vi "Save Config File (to internal memory).vi"(8 "error in (no error)":errorcluster, 10 "Name of the config to store in the DAS":string, 11 "VISA resource name":refnum<visa-resource-name>) -> (0 "error out":errorcluster, 3 "VISA resource name out":refnum<visa-resource-name>)   [LabVIEW 2017, in "Sefram DAS220.lvlib"]
doc: "Save the current configuration into the device internal memory."
uses:
  <instrlib>/Sefram DAS220/Sefram DAS220.lvlib
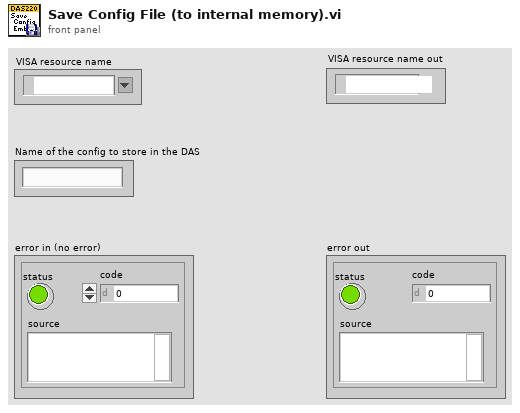
[diagram p1: front panel]
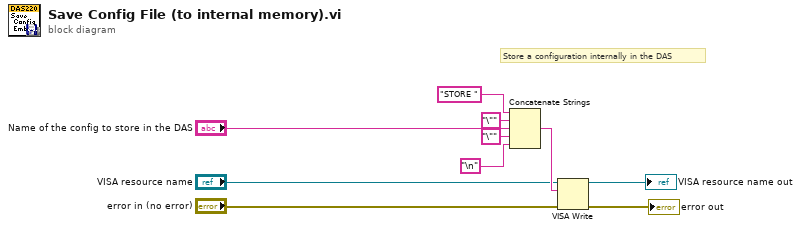
[diagram p0: block diagram]
diagram:
  # "Store a configuration internally in the DAS"
  n1 = Concatenate Strings("STORE " ("string"), "\"" ("string"), "Name of the config to store in the DAS", "\"" ("string"), "\n") -> (w10:string)
  n2 = VISA Write(VISA resource name="VISA resource name", write buffer=w10, error in (no error)="error in (no error)") -> (VISA resource name out=→"VISA resource name out":refnum<visa-resource-name>, error out=→"error out":errorcluster)  [unwired: 1 out]
